vi "Wait Settle Time.vi"(8 "error in (no error)":errorcluster, 11 "Model in":refnum<class "Model.lvclass">) -> (0 "error out":errorcluster, 3 "Model out":refnum<class "Model.lvclass">)   [LabVIEW 2016, in "Model.lvclass"]
uses:
  Model.lvclass
  Model.lvclass/Model.ctl
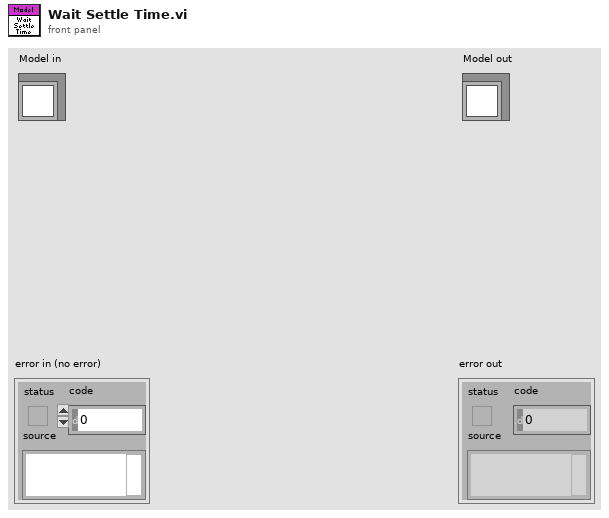
[diagram p1: front panel]
types:
  T1 = typedef "HPMT_Typedefs.lvlib/TestSettings.ctl" = cluster{"Operator":string, "Strut Number":string, "Test Stand Serial Number":string, "Notes":string, "Test Angle":u16, "Number of Cycles":u16, "Data Points per Cycle":u16, "Settling Time (secs)":u16, "Breakaway Air Pressure":u16, "Largest Strut Displacement":dbl, "Load Cell Sensitivity":dbl, "Micron to Step Ratio":dbl, "Micron to Encoder Ratio":dbl}
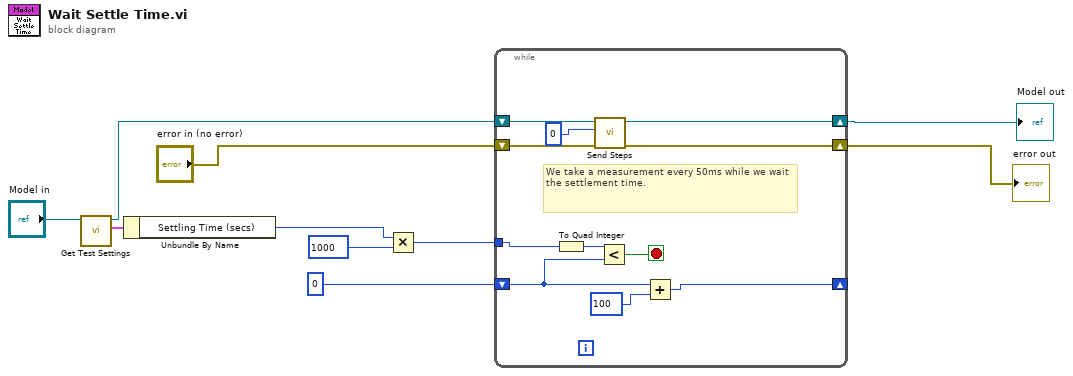
[diagram p0: block diagram]
diagram:
  n1 = call "Get Test Settings.vi"("Model in"="Model in") -> ("Test Settings"=w9:T1, "Model out"=w4:refnum<class "Model.lvclass">)  [unwired: 9 in]
  n2 = Unbundle By Name(w9) -> ("Settling Time (secs)"=w7:u16)
  n3 = Multiply(x=w7, y=u16 1000) -> (x*y=w5:u16)
  n4 = while {
    shift-right: [w21] -> _
    shift-left: i64 0 -> [w19]
    tunnel: w5 -> [w18]
    shift-right: [w13] -> w3
    shift-left: w4 -> [w16]
    shift-right: [w12] -> w1
    shift-left: "error in (no error)" -> [w15]
    stop <- w20 stop-if-true
    # "We take a measurement every 50ms while we wait the settlement time."
    n5 = To Quad Integer(1:w18) -> (0:w17:i64)
    n6 = call "Send Steps.vi"("error in (no error)"=w15, "Command.Steps"=0, "Model in"=w16) -> ("error out"=w12:errorcluster, "Model out"=w13:refnum<class "Model.lvclass">)  [unwired: 7 in]
    n7 = Less?(x=w17, y=w19) -> (x < y?=w20:bool)
    n8 = Add(x=w19, y=i64 100) -> (x+y=w21:i64)
  }
  "error out" <- w1
  "Model out" <- w3
